vi "PDP Log Message.vi"(0 "Message":string) -> ()   [LabVIEW 2010]
uses:
  PDP Global.vi
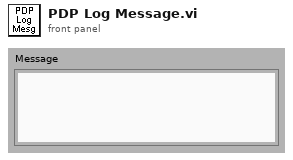
[diagram p1: front panel]
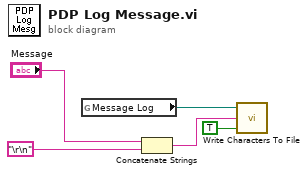
[diagram p0: block diagram]
diagram:
  n1 = global read "PDP Global.vi" "Message Log"() -> (w5:path)
  n2 = Concatenate Strings("Message", "\r\n") -> (w2:string)
  n3 = call <vilib>:"Write Characters To File.vi"("append to file? (new file:F)"=TRUE, "character string"=w2, "file path (dialog if empty)"=w5) -> ()  [unwired: 2 in, 1 out]
